vi "Interface.vi"() -> ()   [LabVIEW 2020]
uses:
  Configs/Type Defs/Config Type Cluster.ctl
  <vilib>/vision/Image Controls.llb/IMAQ Image.ctl
  QHM/QHM.lvlib
  Configs/Settings Manager.lvlib
panel:
  out "Image Out":T1(plugin-control)
  out "Config Control Refnums":T2[](array[typedef])
  in  "Tab Control":enum32{"Configurações", "Câmera"}(tab)
  in  "Salvar configs.":bool
  in  "Tipo de Captura":enum16{"Pasta com Imagens", "Câmera"}(ring)
  in  "Pasta com imagens":path
  in  "Stop":bool
  out "Relógio":timestamp format="%<%x %X>T"
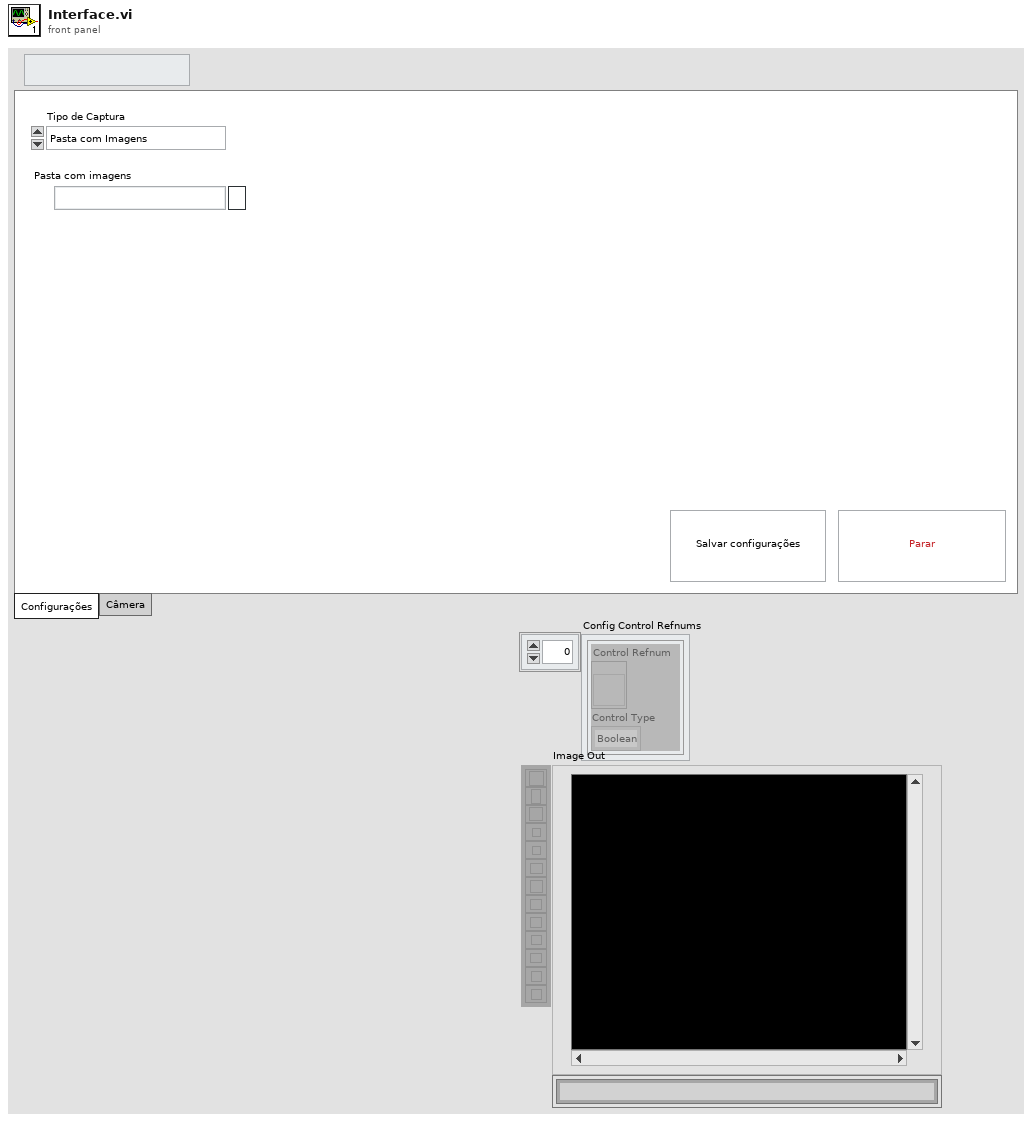
[diagram p1: front panel]
types:
  T1 = typedef "IMAQ Image.ctl" = refnum<image>
  T2 = typedef "Settings Manager.lvlib/Config Type Cluster.ctl" = cluster{"Control Refnum":refnum<vi>, "Control Type":enum16{"Boolean", "String", "Integer", "Float", "Path"}}
  T3 = enum16{"Boolean", "String", "Integer", "Float", "Path"}
  T4 = enum8{"Enabled", "Disabled", "Disabled and Grayed Out"}
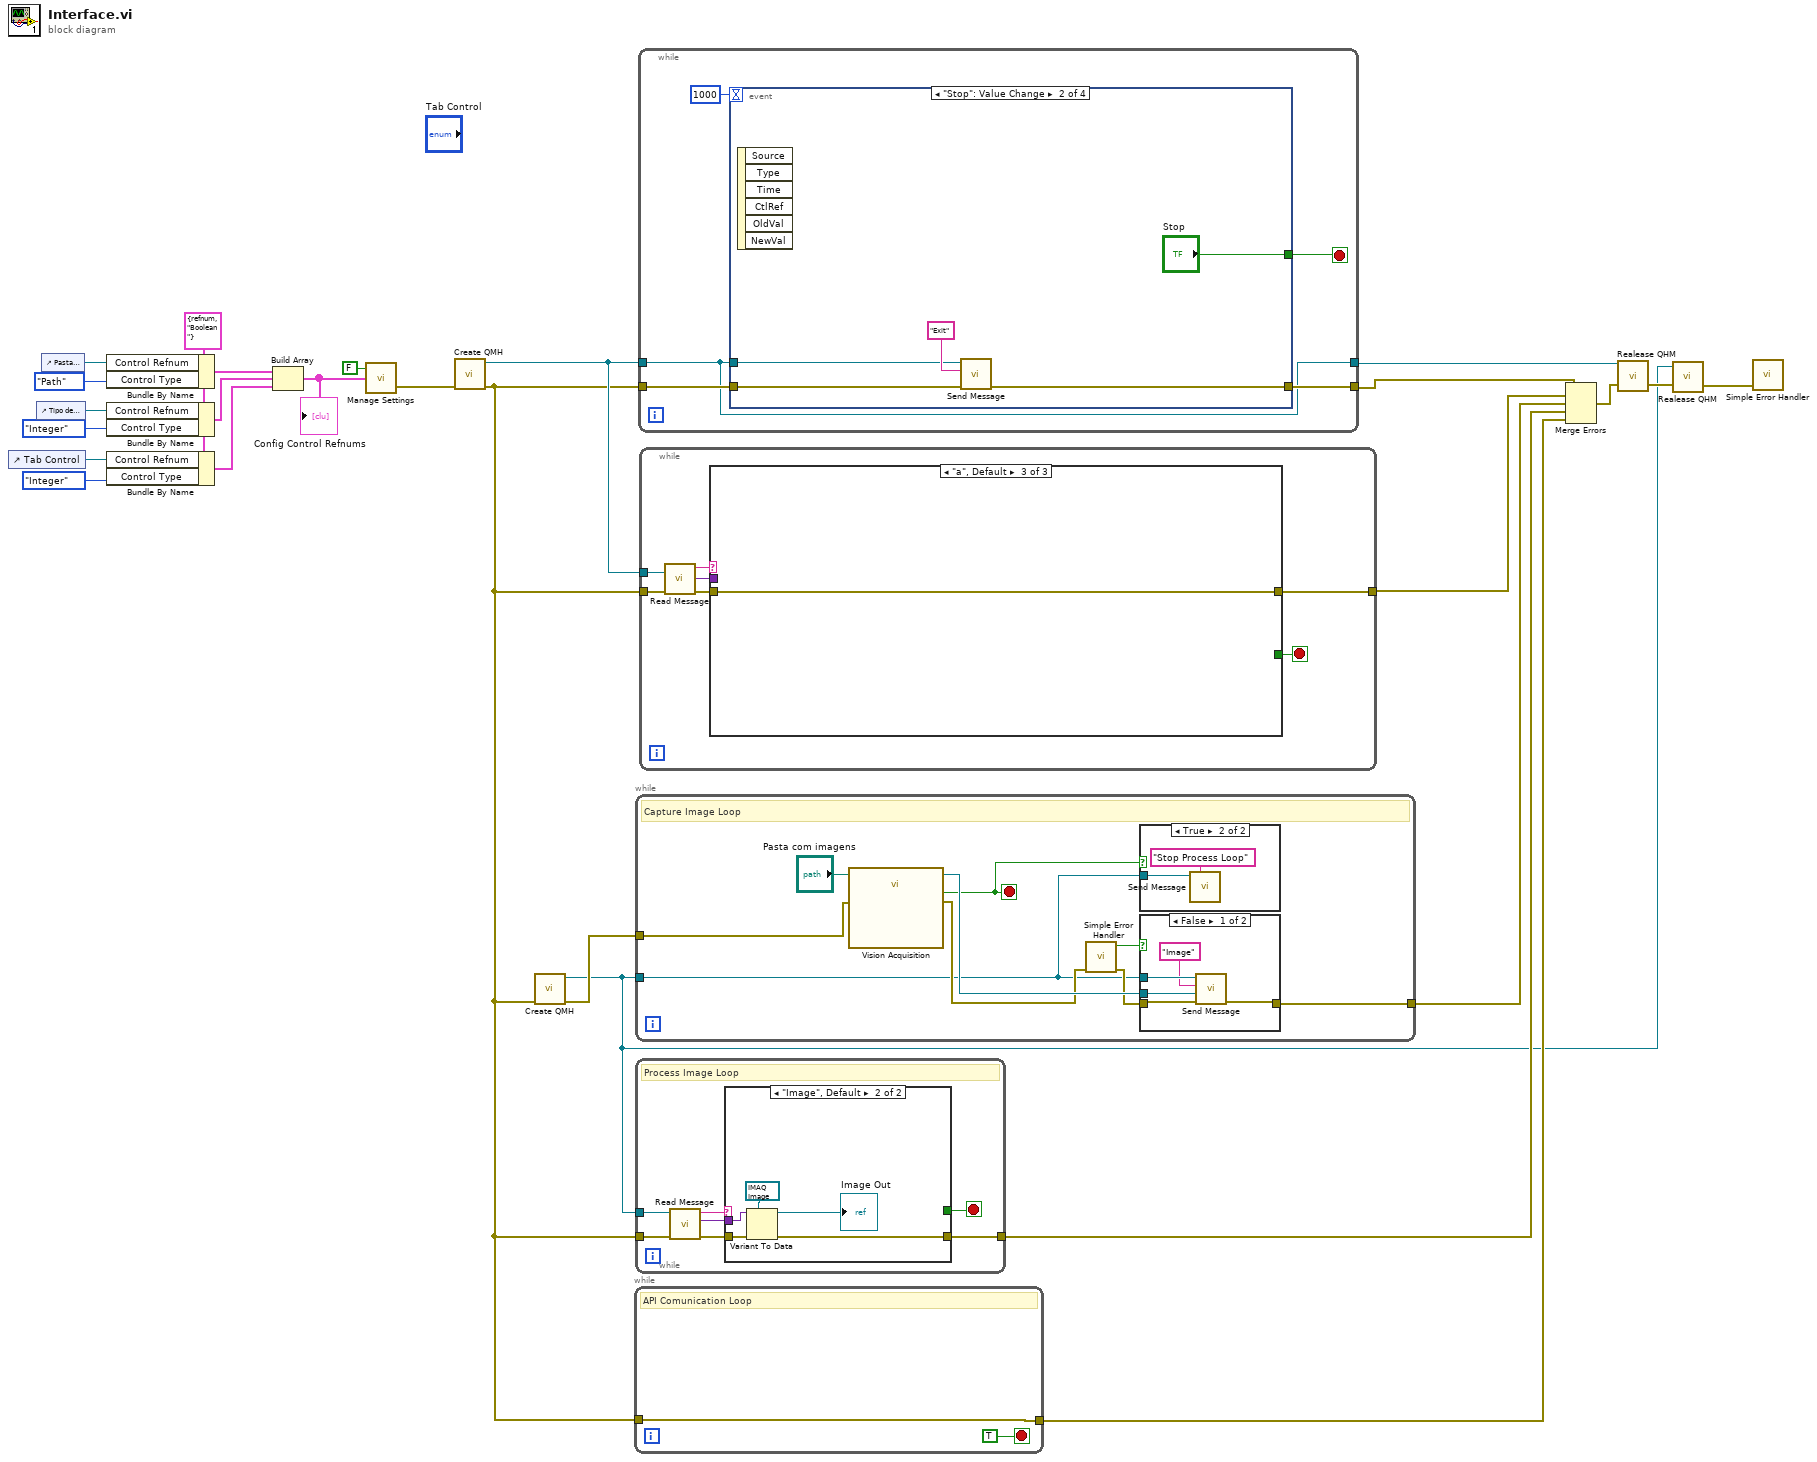
[diagram p0: block diagram]
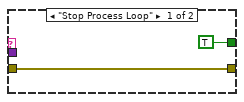
[diagram p2: hidden frame]
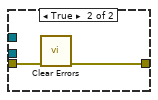
[diagram p4: hidden frame]
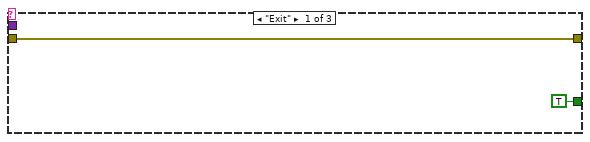
[diagram p5: hidden frame]
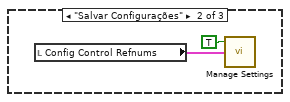
[diagram p6: hidden frame]
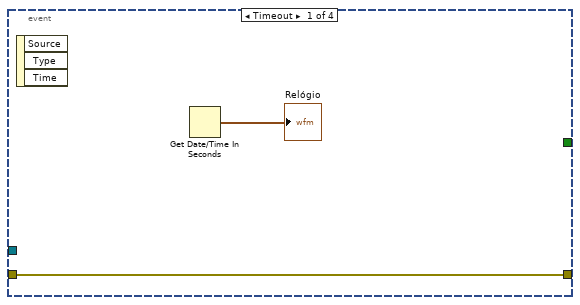
[diagram p7: hidden frame]
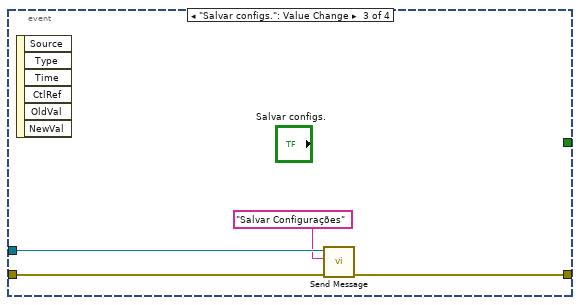
[diagram p8: hidden frame]
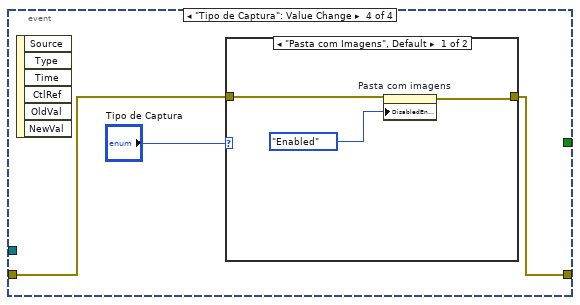
[diagram p9: hidden frame]
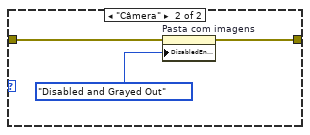
[diagram p10: hidden frame]
diagram:
  w15 = T2 {"Control Refnum"=refnum, "Control Type"=enum."Boolean"} ("input cluster")
  n1 = control-ref of="Tab Control"() -> (w14:refnum<vi>)
  n2 = control-ref of="Tipo de Captura"() -> (w17:refnum<vi>)
  n3 = control-ref of="Pasta com imagens"() -> (w19:refnum<vi>)
  n4 = Bundle By Name(cluster=w15, "Control Refnum"=w19, "Control Type"=T3."Path") -> (w20:T2)
  n5 = Bundle By Name(cluster=w15, "Control Refnum"=w17, "Control Type"=T3."Integer") -> (w12:T2)
  n6 = Bundle By Name(cluster=w15, "Control Refnum"=w14, "Control Type"=T3."Integer") -> (w11:T2)
  n7 = Build Array(w20, w12, w11) -> (w9:T2[])
  "Config Control Refnums" <- w9
  n8 = call "Manage Settings.vi"("Config Cluster Array Input"=w9, "Save Current Values"=FALSE) -> ("error out"=w8:errorcluster)  [unwired: 1 in, 1 out]
  n9 = call "Create QMH.vi"("error in (no error)"=w8) -> ("error out"=w6:errorcluster, "Queue Message Handler"=w7:refnum<queue>)  [unwired: 9 in]
  n10 = call "Create QMH.vi"("error in (no error)"=w6) -> ("error out"=w5:errorcluster, "Queue Message Handler"=w1:refnum<queue>)  [unwired: 9 in]
  n11 = while {
    tunnel: w6 -> [w28]
    tunnel: [w28] -> w21
    stop <- TRUE stop-if-true
    # "API Comunication Loop"
  }
  n12 = while {
    tunnel: w1 -> [w30]
    tunnel: [w36] -> w4
    tunnel: w5 -> [w29]
    stop <- w31 stop-if-true
    # "Capture Image Loop"
    n13 = call "Vision Acquisition"("Image Path"="Pasta com imagens", "error in"=w29) -> ("Image Out"=w35:T1, "Stopped"=w31:bool, "error out"=w32:errorcluster)  [unwired: 22 in, 1 out]
    n14 = call <vilib>:"Simple Error Handler.vi"("error in (no error)"=w32) -> ("error?"=w33:bool, "error out"=w34:errorcluster)  [unwired: 4 in, 3 out]
    n15 = case shown="True" w31 {
      tunnel: w30 -> [_ w39]
      frame False {
      }
      frame True {
        n16 = call "Send Message.vi"("Event"="Stop Process Loop", "Queue in"=w39) -> ()  [unwired: 4 in, 2 out]
      }
    }
    n17 = case shown="False" w33 {
      tunnel: w30 -> [w44 _]
      tunnel: w34 -> [w42 w46]
      tunnel: [w43 w45] -> w36
      tunnel: w35 -> [w41 _]
      frame False {
        n18 = call "Send Message.vi"("error in (no error)"=w42, "Message"=w41, "Event"="Image", "Queue in"=w44) -> ("error out"=w43:errorcluster)  [unwired: 2 in, 1 out]
      }
      frame True {
        n19 = call <vilib>:"Clear Errors.vi"("error in (no error)"=w46) -> ("error out"=w45:errorcluster)  [unwired: 5 in, 1 out]
      }
    }
  }
  n20 = while {
    tunnel: [w50] -> w22
    tunnel: w6 -> [w53]
    tunnel: w1 -> [w52]
    stop <- w47 stop-if-true
    # "Process Image Loop"
    n21 = call "Read Message.vi"("error in (no error)"=w53, "QMH in"=w52) -> ("error out"=w51:errorcluster, "Message"=w48:variant, "Event"=w49:string)  [unwired: 2 in, 1 out]
    n22 = case shown="\"Image\", Default" w49 {
      tunnel: w51 -> [w54 w60]
      tunnel: [w54 w59] -> w50
      tunnel: w48 -> [_ w58]
      tunnel: [TRUE _] -> w47
      frame "Stop Process Loop" {
      }
      frame "Image", Default {
        n23 = Variant To Data(error in=w60, type=T1 refnum ("Image Out"), Variant=w58) -> (data=→"Image Out":T1, error out=w59:errorcluster)
      }
    }
  }
  n24 = while {
    tunnel: w7 -> [w61]
    tunnel: [w61] -> w26
    tunnel: w6 -> [w63]
    tunnel: [w62] -> w23
    stop <- w64 stop-if-true
    n25 = event shown="[1] \"Stop\": Value Change" {
      selector: _ -> [_ _ _ _]
      dyn-events: _ -> [_ _ _ _]
      timeout: 1000 -> [_ _ _ _]
      tunnel: w61 -> [_ w71 w74 _]
      tunnel: [_ "Stop" _ _] -> w64
      tunnel: w63 -> [w66 w69 w76 w78]
      tunnel: [w66 w68 w75 w77] -> w62
      event Timeout {
        n26 = event-data() -> ()  [unwired: 1 in, 3 out]
        n27 = Get Date/Time In Seconds() -> (seconds since 1Jan1904=→"Relógio":timestamp)
      }
      event "Stop": Value Change {
        n28 = event-data() -> ()  [unwired: 1 in, 6 out]
        n29 = call "Send Message.vi"("error in (no error)"=w69, "Event"="Exit", "Queue in"=w71) -> ("error out"=w68:errorcluster)  [unwired: 3 in, 1 out]
      }
      event "Salvar configs.": Value Change {
        n30 = event-data() -> ()  [unwired: 1 in, 6 out]
        n31 = call "Send Message.vi"("error in (no error)"=w76, "Event"="Salvar Configurações", "Queue in"=w74) -> ("error out"=w75:errorcluster)  [unwired: 3 in, 1 out]
      }
      event "Tipo de Captura": Value Change {
        n32 = event-data() -> ()  [unwired: 1 in, 6 out]
        n33 = case shown="\"Pasta com Imagens\", Default" "Tipo de Captura" {
          tunnel: w78 -> [w81 w84]
          tunnel: [w80 w83] -> w77
          frame "Pasta com Imagens", Default {
            n34 = property on="Pasta com imagens" class="Path"(error in=w81, "DisabledEnum"=T4."Enabled" ("Disabled")) -> (error out=w80:errorcluster)  [unwired: 1 in, 1 out]
          }
          frame "Câmera" {
            n35 = property on="Pasta com imagens" class="Path"(error in=w84, "DisabledEnum"=T4."Disabled and Grayed Out" ("Disabled")) -> (error out=w83:errorcluster)  [unwired: 1 in, 1 out]
          }
        }
      }
    }
  }
  n36 = while {
    tunnel: w7 -> [w92]
    tunnel: [w88] -> w24
    tunnel: w6 -> [w87]
    stop <- w90 stop-if-true
    n37 = call "Read Message.vi"("error in (no error)"=w87, "QMH in"=w92) -> ("error out"=w89:errorcluster, "Message"=w86:variant, "Event"=w91:string)  [unwired: 2 in, 1 out]
    n38 = case shown="\"a\", Default" w91 {
      tunnel: [TRUE _ _] -> w90
      tunnel: w89 -> [w93 _ w97]
      tunnel: [w93 _ w97] -> w88
      tunnel: w86 -> [_ _ _]
      frame "Exit" {
      }
      frame "Salvar Configurações" {
        n39 = local read "Config Control Refnums"() -> (w96:T2[])
        n40 = call "Manage Settings.vi"("Config Cluster Array Input"=w96, "Save Current Values"=TRUE) -> ()  [unwired: 1 in, 2 out]
      }
      frame "a", Default {
      }
    }
  }
  n41 = Merge Errors(w23, w24, w4, w22, w21) -> (w25:errorcluster)
  n42 = call "Realease QHM.vi"("error in (no error)"=w25, "QHM in"=w26) -> ("error out"=w3:errorcluster)  [unwired: 1 in]
  n43 = call "Realease QHM.vi"("error in (no error)"=w3, "QHM in"=w1) -> ("error out"=w2:errorcluster)  [unwired: 1 in]
  n44 = call <vilib>:"Simple Error Handler.vi"("error in (no error)"=w2) -> ()  [unwired: 4 in, 5 out]
